vi "Is GigE Vision.vi"(8 "error in (no error)":errorcluster, 11 "Camera in":refnum<class "Camera.lvclass">) -> (0 "error out":errorcluster, 2 "Is GigE Vision":bool, 3 "Camera":refnum<class "Camera.lvclass">)   [LabVIEW 2020, in "Camera.lvclass"]
uses:
  Camera.lvclass
  Camera.lvclass/Camera.ctl
  bin/gindustrialcam_32-1.dll
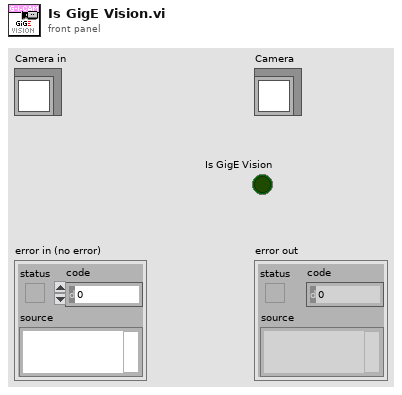
[diagram p1: front panel]
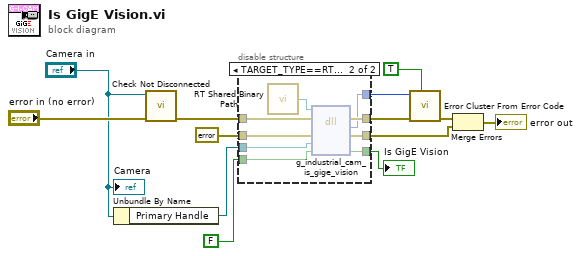
[diagram p0: block diagram]
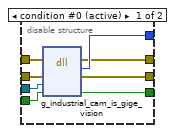
[diagram p2: hidden frame]
diagram:
  n1 = Unbundle By Name("Camera in") -> ("Primary Handle"=w3:refnum<data-value>)
  n2 = call "Check Not Disconnected.vi"("error in (no error)"="error in (no error)", "Camera in"="Camera in") -> ("error out"=w11:errorcluster)  [unwired: 9 in]
  n3 = disable-structure shown="TARGET_TYPE==RT&&OS==Linux" {
    disable-tunnel: w11 -> [w21 w30]
    disable-tunnel: errorcluster {"status"=FALSE, "code"=0, "source"=""} ("error constant") -> [w20 w27]
    disable-tunnel: [w19 w23] -> w8
    disable-tunnel: [w18 w28] -> w6
    disable-tunnel: [w17 w29] -> w5
    disable-tunnel: w3 -> [w16 w26]
    disable-tunnel: FALSE -> [w15 w25]
    disable-tunnel: [w14 w24] -> w1
    frame condition #0 (active) {
      n4 = dll-call lib="C:/serenial/lib/g-industrial-camera/LabVIEW/g_industrial_cam/bin/gindustrialcam_*-1.*" fn="g_industrial_cam_is_gige_vision"(error in=w21, "err"=w20, "edvr"=w16, "boolean"=w15) -> (error out=w17:errorcluster, "Mg_Error"=w18:i32, "err"=w19:errorcluster, "boolean"=w14:bool)  [unwired: 3 in, 1 out]
    }
    frame condition #1 {
      n5 = call "RT Shared Binary Path.vi"() -> ("Path"=w22:path)
      n6 = dll-call lib="?" fn="g_industrial_cam_is_gige_vision"(path in=w22, error in=w30, "err"=w27, "edvr"=w26, "boolean"=w25) -> (error out=w29:errorcluster, "Mg_Error"=w28:i32, "err"=w23:errorcluster, "boolean"=w24:bool)  [unwired: 2 in, 1 out]
    }
  }
  "Is GigE Vision" <- w1
  n7 = call <vilib>:"Error Cluster From Error Code.vi"("show call chain? (False)"=TRUE, "error in (no error)"=w5, "error code (0)"=w6) -> ("error out"=w7:errorcluster)  [unwired: 6 in]
  n8 = Merge Errors(w7, w8) -> (→"error out":errorcluster)
  "Camera" <- "Camera in"
